vi "get_cluster_labels.vi"(1 "Conditions cluster":T1) -> (0 "Lables":string[](array[string]))   [LabVIEW 2019]
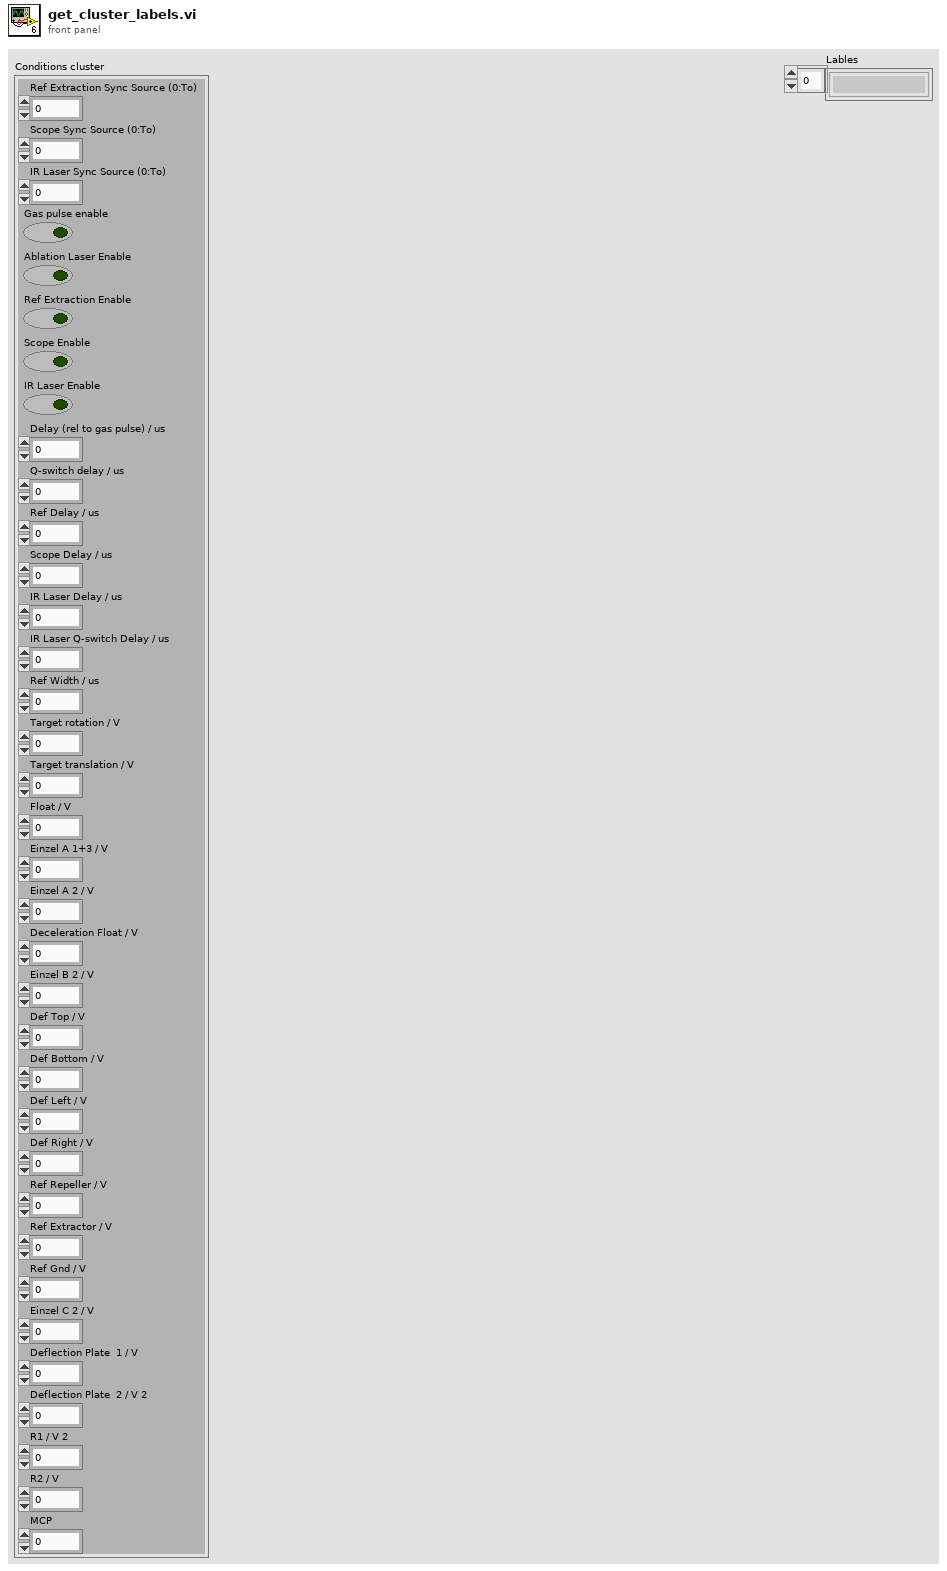
[diagram p1: front panel]
types:
  T1 = cluster{"Ref Extraction Sync Source (0:To)":i32, "Scope Sync Source (0:To)":i32, "IR Laser Sync Source (0:To)":i32, "Gas pulse enable":bool, "Ablation Laser Enable":bool, "Ref Extraction Enable":bool, "Scope Enable":bool, "IR Laser Enable":bool, "Delay (rel to gas pulse) / us":dbl, "Q-switch delay / us":dbl, "Ref Delay / us":dbl, "Scope Delay / us":dbl, "IR Laser Delay / us":dbl, "IR Laser Q-switch Delay / us":dbl, "Ref Width / us":dbl, "Target rotation / V":dbl, "Target translation / V":dbl, "Float / V":dbl, "Einzel A 1+3 / V":dbl, "Einzel A 2 / V":dbl, "Deceleration Float / V":dbl, "Einzel B 2 / V":dbl, "Def Top / V":dbl, "Def Bottom / V":dbl, "Def Left / V":dbl, "Def Right / V":dbl, "Ref Repeller / V":dbl, "Ref Extractor / V ":dbl, "Ref Gnd / V ":dbl, "Einzel C 2 / V":dbl, "Deflection Plate  1 / V":dbl, "Deflection Plate  2 / V 2":dbl, "R1 / V 2":dbl, "R2 / V":dbl, "MCP":dbl}
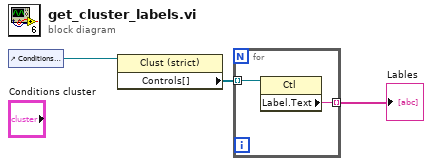
[diagram p0: block diagram]
diagram:
  n1 = control-ref of="Conditions cluster"() -> (w3:refnum<vi>)
  n2 = property class="Clust (strict)"(reference=w3) -> ("Controls[]"=w2:refnum<vi>[])  [unwired: 1 in, 2 out]
  n3 = for {
    tunnel: w2 -> [w5] mode=indexing
    tunnel: [w4] -> w1 mode=indexing
    n4 = property class="Ctl"(reference=w5) -> ("Label.Text"=w4:string)  [unwired: 1 in, 2 out]
  }
  "Lables" <- w1
